vi "instance count allowed.vi"(8 "error in":errorcluster, 11 "dds configuration in":refnum<class "dds configuration.lvclass">) -> (0 "error out":errorcluster, 2 "instances allowed":i32, 3 "dds configuration out":refnum<class "dds configuration.lvclass">)   [LabVIEW 2020, in "DDS configuration.lvclass"]
uses:
  dds configuration.lvclass
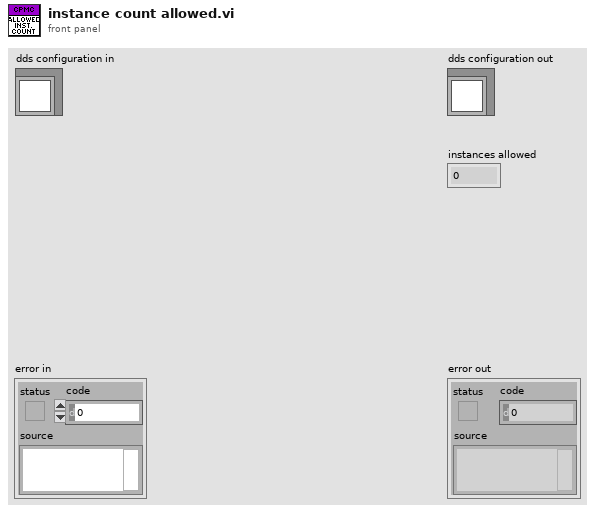
[diagram p1: front panel]
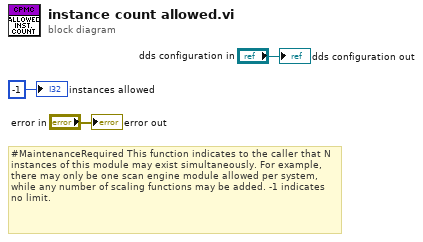
[diagram p0: block diagram]
diagram:
  # "#MaintenanceRequired This function indicates to the caller that N instances of this module may exist simultaneously. For example, there may only be one scan engine module allowed per system, while any number of scaling functions may be added. -1 indicates no limit."
  "error out" <- "error in"
  "dds configuration out" <- "dds configuration in"
  "instances allowed" <- -1 ("instances allowed")
